vi "set PG according to private data.vi"(8 "error in (no error)":errorcluster, 11 "Pulse Gen Scan in":refnum<class "Pulse Gen Scan.lvclass">) -> (0 "error out":errorcluster, 3 "Pulse Gen Scan out":refnum<class "Pulse Gen Scan.lvclass">)   [LabVIEW 2012, in "Pulse Gen Scan.lvclass"]
uses:
  Pulse Gen Scan.lvclass
  Pulse Gen Scan.lvclass/Pulse Gen Scan.ctl
  Instruments/Utility Classes/Scannable/Scannable.lvclass
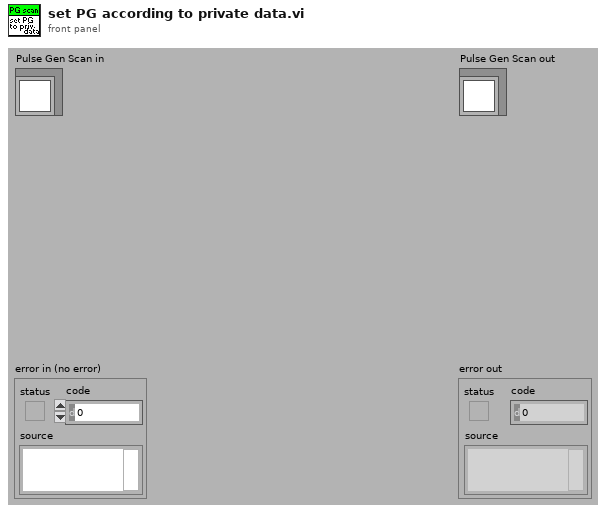
[diagram p1: front panel]
types:
  T1 = enum16{"Channel All ", "Channel 1", "Channel 2", "Channel 3", "Channels Combined"}
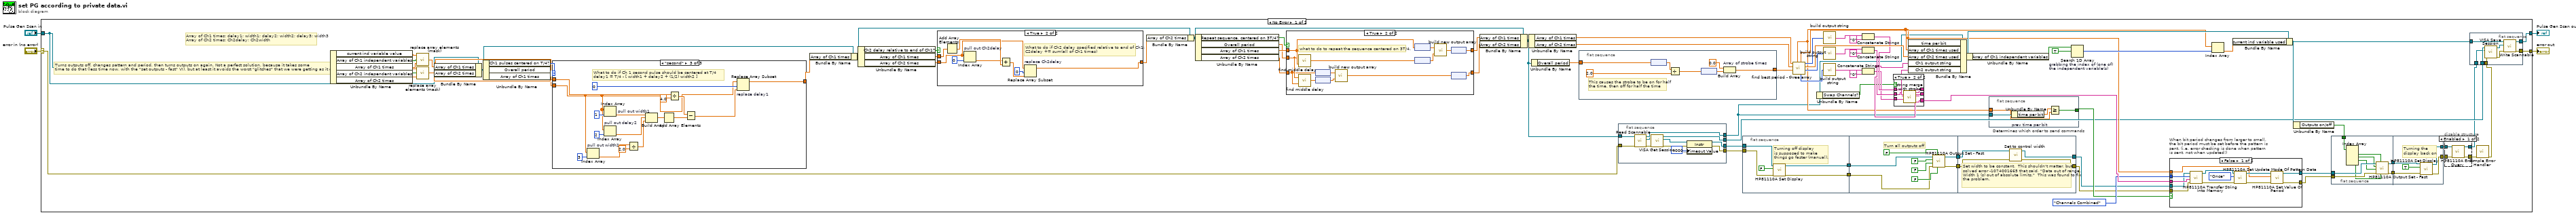
[diagram p0: block diagram]
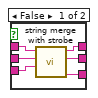
[diagram p2: hidden frame]
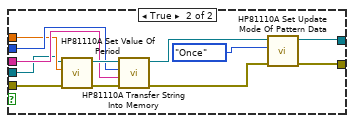
[diagram p3: hidden frame]
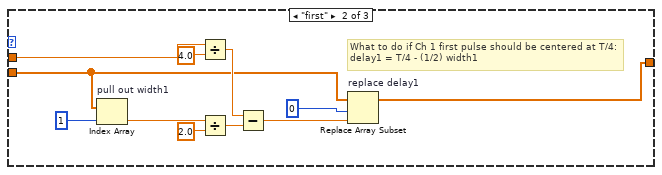
[diagram p7: hidden frame]
diagram:
  n1 = case shown="No Error" "error in (no error)" {
    selector: "error in (no error)" -> [w51 w242]
    tunnel: [w50 w242] -> w3
    tunnel: "Pulse Gen Scan in" -> [w73 w241]
    tunnel: [w49 w241] -> w1
    frame No Error {
      # "Turns outputs off, changes pattern and period, then turns outputs on again. Not a perfect solution, because it takes some \ntime to do that (less time now, with the \"set outputs - fast\" VI), but at least it avoids the worst \"glitches\" that we were getting as it changed pts."
      # "Array of Ch1 times: delay1; width1; delay2; width2; delay3; width3\nArray of Ch2 times: Ch2delay; Ch2width"
      n2 = Unbundle By Name(w73) -> ("current ind variable value"=w72:dbl[unit], "Array of Ch1 independent variables"=w78:bool[], "Array of Ch1 times"=w77:dbl[unit][], "Array of Ch2 independent variables"=w71:bool[], "Array of Ch2 times"=w70:dbl[unit][])
      n3 = call "replace array elements (mask).vi"("input array of numbers"=w77, "array of booleans (mask)"=w78, "value"=w72) -> ("output array"=w74:dbl[unit][])
      n4 = call "replace array elements (mask).vi"("input array of numbers"=w70, "array of booleans (mask)"=w71, "value"=w72) -> ("output array"=w69:dbl[unit][])
      n5 = Bundle By Name(cluster=w73, "Array of Ch1 times"=w74, "Array of Ch2 times"=w69) -> (w67:refnum<class "Pulse Gen Scan.lvclass">)
      n6 = Unbundle By Name(w67) -> ("Ch1 pulses centered on T/4?"=w81:enum32{"none", "first", "second"}, "Overall period"=w76:dbl[unit], "Array of Ch1 times"=w75:dbl[unit][])
      n7 = case shown="\"second\"" w81 {
        tunnel: w75 -> [w197 w199 w211]
        tunnel: [w197 w201 w217] -> w68
        tunnel: w76 -> [_ w202 w218]
        frame "none", Default {
        }
        frame "first" {
          # "What to do if Ch 1 first pulse should be centered at T/4:\ndelay1 = T/4 - (1/2) width1"
          n8 = Index Array "pull out width1"(array=w199, index=1) -> (element=w198:dbl[unit])
          n9 = Divide(x=w202, y=4.0) -> (x/y=w207:dbl[unit])
          n10 = Divide(x=w198, y=2.0) -> (x/y=w205:dbl[unit])
          n11 = Subtract(x=w207, y=w205) -> (x-y=w203:dbl[unit])
          n12 = Replace Array Subset "replace delay1"(array=w199, new element=w203, index=0) -> (w201:dbl[unit][])
        }
        frame "second" {
          # "What to do if Ch 1 second pulse should be centered at T/4\ndelay1 = T/4 - [ width1 + delay2 + (1/2) width2 ]"
          n13 = Index Array "pull out width2"(array=w211, index=3) -> (element=w210:dbl[unit])
          n14 = Index Array "pull out width1"(array=w211, index=1) -> (element=w215:dbl[unit])
          n15 = Index Array "pull out delay2"(array=w211, index=2) -> (element=w213:dbl[unit])
          n16 = Divide(x=w210, y=2.0) -> (x/y=w220:dbl[unit])
          n17 = Build Array(w215, w213, w220) -> (w222:dbl[unit][])
          n18 = Add Array Elements(numeric array=w222) -> (sum=w221:dbl[unit])
          n19 = Divide(x=w218, y=4.0) -> (x/y=w224:dbl[unit])
          n20 = Subtract(x=w224, y=w221) -> (x-y=w209:dbl[unit])
          n21 = Replace Array Subset "replace delay1"(array=w211, new element=w209, index=0) -> (w217:dbl[unit][])
        }
      }
      n22 = Bundle By Name(cluster=w67, "Array of Ch1 times"=w68) -> (w52:refnum<class "Pulse Gen Scan.lvclass">)
      n23 = Unbundle By Name(w52) -> ("Ch2 delay relative to end of Ch1?"=w62:bool, "Array of Ch1 times"=w66:dbl[unit][], "Array of Ch2 times"=w61:dbl[unit][])
      n24 = case shown="True" w62 {
        tunnel: [w188 w191] -> w65
        tunnel: w61 -> [w188 w189]
        tunnel: w66 -> [_ w195]
        frame False {
        }
        frame True {
          # "What to do if Ch2 delay specified relative to end of Ch1:\nC2delay += sum(all of Ch1 times)"
          n25 = Add Array Elements(numeric array=w195) -> (sum=w196:dbl[unit])
          n26 = Index Array "pull out Ch2delay"(array=w189, index=0) -> (element=w190:dbl[unit])
          n27 = Add(x=w190, y=w196) -> (x+y=w192:dbl[unit])
          n28 = Replace Array Subset "replace Ch2delay"(array=w189, new element=w192, index=0) -> (w191:dbl[unit][])
        }
      }
      n29 = Bundle By Name(cluster=w52, "Array of Ch2 times"=w65) -> (w58:refnum<class "Pulse Gen Scan.lvclass">)
      n30 = Unbundle By Name(w58) -> ("Repeat sequence, centered on 3T/4?"=w59:bool, "Overall period"=w60:dbl[unit], "Array of Ch1 times"=w63:dbl[unit][], "Array of Ch2 times"=w64:dbl[unit][])
      n31 = case shown="True" w59 {
        tunnel: w63 -> [w227 w234]
        tunnel: [w227 w237] -> w57
        tunnel: w64 -> [w226 w229]
        tunnel: [w226 w235] -> w56
        tunnel: w60 -> [_ w232]
        frame False {
        }
        frame True {
          # "what to do to repeat the sequence centered on 3T/4."
          n32 = call "find middle delay.vi"("array of times"=w234, "Expected overall period"=w232) -> ("middle delay"=w233:dbl[unit])
          n33 = call "find middle delay.vi"("array of times"=w229, "Expected overall period"=w232) -> ("middle delay"=w231:dbl[unit])
          n34 = node(w229) -> (w228:dbl[])
          n35 = node(w231) -> (w230:dbl)
          n36 = call "build new output array.vi"("number to insert"=w230, "input array"=w228) -> ("output array"=w236:dbl[])
          n37 = node(w234) -> (w240:dbl[])
          n38 = node(w233) -> (w239:dbl)
          n39 = call "build new output array.vi"("number to insert"=w239, "input array"=w240) -> ("output array"=w238:dbl[])
          n40 = node(w238) -> (w237:dbl[unit][])
          n41 = node(w236) -> (w235:dbl[unit][])
        }
      }
      n42 = Bundle By Name(cluster=w58, "Array of Ch1 times"=w57, "Array of Ch2 times"=w56) -> (w36:refnum<class "Pulse Gen Scan.lvclass">)
      n43 = Unbundle By Name(w36) -> ("Array of Ch1 times"=w44:dbl[unit][], "Array of Ch2 times"=w43:dbl[unit][])
      n44 = Unbundle By Name(w36) -> ("Overall period"=w35:dbl[unit])
      n45 = flat-sequence {
        tunnel: [w147] -> w42
        tunnel: w35 -> [w146]
        frame #0 {
          # "This causes the strobe to be on for half the time, then off for half the time"
          n46 = node(w146) -> (w150:dbl)
          n47 = Divide(x=w150, y=2.0) -> (x/y=w148:dbl)
          n48 = node(w148) -> (w145:dbl[unit])
          n49 = Build Array "Array of strobe times"(dbl[unit] 0.0 ("element"), w145) -> (w147:dbl[unit][])
        }
      }
      n50 = flat-sequence {
        tunnel: w51 -> [w119]
        tunnel: [w118] -> w11
        tunnel: [w117] -> w48
        tunnel: [w116] -> w47
        tunnel: w36 -> [w115]
        tunnel: [w114] -> w8
        frame #0 {
          n51 = call-dynamic "Read Scannable.vi"("error in (no error)"=w119, "Scanner.lvclass in"=w115) -> ("error out"=w112:errorcluster, "Scannable.lvclass"=w113:refnum<class "Scannable.lvclass">, "Scanner.lvclass out"=w114:refnum<class "Pulse Gen Scan.lvclass">)  [unwired: 7 out]
          n52 = call-dynamic "VISA Get Session.vi"("error in (no error)"=w112, "Instrument.lvclass in"=w113) -> ("error out"=w109:errorcluster, "VISA Resource Name"=w110:refnum<visa-resource-name>, "Instrument.lvclass out"=w118:refnum<class "Scannable.lvclass">)  [unwired: 6 in, 1 out]
          n53 = property class="Instr"(reference=w110, error in=w109, "General Settings:Timeout Value"=u32 4000) -> (reference out=w117:refnum<visa-resource-name>, error out=w116:errorcluster)
        }
      }
      n54 = flat-sequence {
        tunnel: w48 -> [w168]
        tunnel: w47 -> [w166]
        tunnel: [w167] -> w15
        tunnel: [w165] -> w14
        tunnel: w15 -> [w173]
        tunnel: w14 -> [w172]
        tunnel: [w171] -> w6
        tunnel: [w170] -> w5
        tunnel: [w179] -> w12
        tunnel: [w178] -> w13
        tunnel: w6 -> [w181]
        tunnel: w5 -> [w180]
        frame #0 {
          # "Turning off display\nis supposed to make \nthings go faster (manual)."
          n55 = call "HP81110A Set Display.vi"("error in (no error)"=w166, "Display (F:Off)"=FALSE, "VISA session"=w168) -> ("error out"=w165:errorcluster, "dup VISA session"=w167:refnum<visa-resource-name>)  [unwired: 7 out]
        }
        frame #1 {
          # "Turn all outputs off"
          n56 = call "HP81110A Output Set - Fast.vi"("notoutput2"=FALSE, "output1"=FALSE, "error in (no error)"=w172, "output2"=FALSE, "notoutput1"=FALSE, "VISA session"=w173) -> ("error out"=w171:errorcluster, "dup VISA session"=w170:refnum<visa-resource-name>)  [unwired: 4 out]
        }
        frame #2 {
          # "Set width to be constant.  This shouldn't matter, but it solved error -1074001665 that said, \"Data out of range. Width 1 (s) out of absolute limits.\"  This was found to fix the problem."
          n57 = call "Set to control width.vi"("error in (no error)"=w181, "VISA session"=w180) -> ("error out"=w178:errorcluster, "dup VISA session"=w179:refnum<visa-resource-name>)  [unwired: 8 in]
        }
      }
      n58 = call "find best period - three array.vi"("Array of strobe desired times"=w42, "Array of Ch2 desired times"=w43, "Array of Ch1 desired times"=w44) -> ("Array of Ch2 \"period-units\""=w38:i32[], "Array of Ch2 actual times"=w39:dbl[unit][], "Array of Ch1 \"period-units\""=w40:i32[], "Array of strobe \"period-units\""=w37:i32[], "Array of Ch1 actual times"=w41:dbl[unit][], "best period"=w21:dbl[unit])  [unwired: 2 in, 1 out]
      n59 = Unbundle By Name(w8) -> ("Swap Channels?"=w7:bool)
      n60 = call "build output string.vi"("Array of \"period-units\""=w40) -> ("output string"=w31:string)
      n61 = call "build output string.vi"("Array of \"period-units\""=w38) -> ("output string"=w30:string)
      n62 = call "build output string.vi"("Array of \"period-units\""=w37) -> ("output string"=w29:string)
      n63 = Concatenate Strings(w31, "0" ("string")) -> (w28:string)
      n64 = Concatenate Strings(w30, "0" ("string")) -> (w27:string)
      n65 = Concatenate Strings(w29, "0" ("string")) -> (w26:string)
      n66 = case shown="True" w7 {
        tunnel: [w87 w96] -> w54
        tunnel: [w86 w95] -> w53
        tunnel: w28 -> [w90 w92]
        tunnel: w27 -> [w89 w91]
        tunnel: w26 -> [w88 w94]
        tunnel: [w85 w93] -> w24
        frame False {
          n67 = call "string merge with strobe.vi"("Strobe String"=w88, "Ch2 String"=w89, "Ch1 String"=w90) -> ("Merged Output String"=w85:string, "Ch2 Output String"=w86:string, "Ch1 Output String"=w87:string)  [unwired: 5 in, 1 out]
        }
        frame True {
          n68 = call "string merge with strobe.vi"("Strobe String"=w94, "Ch2 String"=w92, "Ch1 String"=w91) -> ("Merged Output String"=w93:string, "Ch2 Output String"=w95:string, "Ch1 Output String"=w96:string)  [unwired: 5 in, 1 out]
        }
      }
      n69 = Bundle By Name(cluster=w8, "time per bit"=w21, "Array of Ch1 times used"=w41, "Array of Ch2 times used"=w39, "Ch1 output string"=w54, "Ch2 output string"=w53) -> (w55:refnum<class "Pulse Gen Scan.lvclass">)
      n70 = Unbundle By Name(w55) -> ("Array of Ch1 independent variables"=w83:bool[])
      n71 = flat-sequence "Determines which order to send commands" {
        tunnel: w8 -> [w108]
        tunnel: [w106] -> w22
        tunnel: w21 -> [w105]
        frame #0 {
          n72 = Unbundle By Name "prev time per bit"(w108) -> ("time per bit"=w107:dbl[unit])
          n73 = Greater Or Equal?(x=w107, y=w105) -> (x >= y?=w106:bool)
        }
      }
      n74 = Search 1D Array "grabbing the index of (one of) \nthe independent variable(s)"(1D array=w83, element=TRUE) -> (index of element=w82:i32)  [unwired: 1 out]
      n75 = case "When bit period changes from larger to small,\nthe bit period must be set before the pattern is\nsent. (i.e. error checking is done when pattern\nis sent, not when updated!)" shown="False" w22 {
        tunnel: [w129 w141] -> w19
        tunnel: [w127 w142] -> w16
        tunnel: w24 -> [w125 w138]
        tunnel: T1."Channels Combined" ("Channel (1:Channel 1)") -> [w126 w135]
        tunnel: w21 -> [w122 w134]
        tunnel: w12 -> [w121 w133]
        tunnel: w13 -> [w120 w132]
        frame False {
          n76 = call "HP81110A Transfer String Into Memory.vi"("error in (no error)"=w120, "String"=w125, "Channel (1:Channel 1)"=w126, "VISA session"=w121) -> ("error out"=w123:errorcluster, "dup VISA session"=w124:refnum<visa-resource-name>)  [unwired: 6 out]
          n77 = call "HP81110A Set Update Mode Of Pattern Data.vi"("error in (no error)"=w123, "Pattern Update Mode (1:Continuous)"=enum16{"Off", "Continuous", "Once"}."Once", "VISA session"=w124) -> ("error out"=w128:errorcluster, "dup VISA session"=w130:refnum<visa-resource-name>)  [unwired: 7 out]
          n78 = call "HP81110A Set Value Of Period.vi"("error in (no error)"=w128, "Period Value"=w122, "VISA session"=w130) -> ("error out"=w127:errorcluster, "dup VISA session"=w129:refnum<visa-resource-name>)  [unwired: 7 out]
        }
        frame True {
          n79 = call "HP81110A Set Value Of Period.vi"("error in (no error)"=w132, "Period Value"=w134, "VISA session"=w133) -> ("error out"=w139:errorcluster, "dup VISA session"=w140:refnum<visa-resource-name>)  [unwired: 7 out]
          n80 = call "HP81110A Transfer String Into Memory.vi"("error in (no error)"=w139, "String"=w138, "Channel (1:Channel 1)"=w135, "VISA session"=w140) -> ("error out"=w136:errorcluster, "dup VISA session"=w137:refnum<visa-resource-name>)  [unwired: 6 out]
          n81 = call "HP81110A Set Update Mode Of Pattern Data.vi"("error in (no error)"=w136, "Pattern Update Mode (1:Continuous)"=enum16{"Off", "Continuous", "Once"}."Once", "VISA session"=w137) -> ("error out"=w142:errorcluster, "dup VISA session"=w141:refnum<visa-resource-name>)  [unwired: 7 out]
        }
      }
      n82 = Index Array(array=w41, index=w82) -> (element=w80:dbl[unit])
      n83 = Bundle By Name(cluster=w55, "current ind variable used"=w80) -> (w25:refnum<class "Pulse Gen Scan.lvclass">)
      n84 = Unbundle By Name(w25) -> ("Outputs on/off"=w20:bool[])
      n85 = flat-sequence {
        tunnel: w20 -> [w159]
        tunnel: w19 -> [w158]
        tunnel: [w157] -> w18
        tunnel: [w156] -> w17
        tunnel: w16 -> [w155]
        tunnel: [w163] -> w46
        tunnel: [w162] -> w45
        tunnel: w18 -> [w161]
        tunnel: w17 -> [w160]
        frame #0 {
          n86 = Index Array(array=w159) -> (element #1=w154:bool, element #2=w153:bool, element #3=w152:bool, element #4=w151:bool)  [unwired: 4 in]
          n87 = call "HP81110A Output Set - Fast.vi"("notoutput2"=w151, "output1"=w154, "error in (no error)"=w155, "output2"=w152, "notoutput1"=w153, "VISA session"=w158) -> ("error out"=w156:errorcluster, "dup VISA session"=w157:refnum<visa-resource-name>)  [unwired: 4 out]
        }
        frame #1 {
          # "Turning the \ndisplay back on"
          n88 = call "HP81110A Set Display.vi"("error in (no error)"=w160, "Display (F:Off)"=TRUE, "VISA session"=w161) -> ("error out"=w162:errorcluster, "dup VISA session"=w163:refnum<visa-resource-name>)  [unwired: 7 out]
        }
      }
      n89 = disable-structure shown="Enabled" {
        disable-tunnel: [w185 w187] -> w79
        disable-tunnel: w46 -> [w184 w186]
        disable-tunnel: w45 -> [w183 w187]
        disable-tunnel: [w182 w186] -> w10
        frame Enabled {
          n90 = call "HP81110A Error Query.vi"("VISA session"=w184, "error in (no error)"=w183) -> ("dup VISA session"=w182:refnum<visa-resource-name>, "error out"=w185:errorcluster)  [unwired: 12 out]
        }
        frame Disabled {
        }
      }
      n91 = flat-sequence {
        tunnel: [w104] -> w50
        tunnel: [w103] -> w49
        tunnel: w25 -> [w102]
        tunnel: w11 -> [w101]
        tunnel: w10 -> [w98]
        tunnel: w9 -> [w97]
        frame #0 {
          n92 = call-dynamic "VISA Save Session.vi"("error in (no error)"=w97, "VISA Resource Name"=w98, "Instrument.lvclass in"=w101) -> ("error out"=w99:errorcluster, "Instrument.lvclass out"=w100:refnum<class "Scannable.lvclass">)  [unwired: 7 out]
          n93 = call-dynamic "Write Scannable.vi"("error in (no error)"=w99, "Scannable.lvclass"=w100, "Scanner.lvclass in"=w102) -> ("error out"=w104:errorcluster, "Scanner.lvclass out"=w103:refnum<class "Pulse Gen Scan.lvclass">)  [unwired: 7 out]
        }
      }
      n94 = call <vilib>:"Simple Error Handler.vi"("error in (no error)"=w79) -> ("error out"=w9:errorcluster)  [unwired: 1 in, 7 out]
    }
    frame Error {
    }
  }
  "error out" <- w3
  "Pulse Gen Scan out" <- w1
